vi "Get Core Group Settings.vi"(8 "error in (no error)":errorcluster, 11 "Item Ref in":T5 format="%.0x") -> (0 "error out":errorcluster, 2 "group configuration":T1={"name"="Group", "direction"=enum."Tx", "cycle timing"={"priority"=100, "decimation"=1, "offset"=0}, "timeout behavior"=enum."Increment Late Count", "enable conversion"=FALSE}, 3 "Item Ref out":T5 format="%.0x")   [LabVIEW 2017, in "DSF Shared.lvlib"]
uses:
  DSF Shared.lvlib
  <vilib>/NI Veristand/Custom Device API/Custom Device Item Ref.ctl
  DSF Core.lvlibp/Typedefs/Core Group Configuration.ctl
  DSF Core.lvlibp/Typedefs/DSF Direction.ctl
  DSF Core.lvlibp/Typedefs/DSF Timing Info.ctl
  DSF Core.lvlibp/Typedefs/DSF Timeout Behavior.ctl
  <vilib>/NI Veristand/Custom Device API/Get Item Property (Variant).vi
  <vilib>/NI Veristand/Custom Device API/Custom Device API.lvlib
  DSF Core.lvlibp
  DSF Core.lvlibp/Classes/Configuration/Core/Group/Group Configuration.lvclass
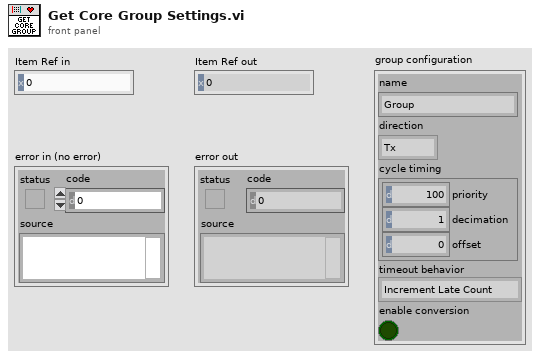
[diagram p1: front panel]
types:
  T1 = typedef "DSF Core.lvlibp/Group Configuration.lvclass/Core Group Configuration.ctl" = cluster{"name":string, "direction":T2, "cycle timing":T3, "timeout behavior":T4, "enable conversion":bool}
  T2 = typedef "DSF Core.lvlibp/DSF Direction.ctl" = enum8{"Tx", "Rx"}
  T3 = typedef "DSF Core.lvlibp/DSF Timing Info.ctl" = cluster{"priority":u64, "decimation":u64, "offset":u64}
  T4 = typedef "DSF Core.lvlibp/DSF Timeout Behavior.ctl" = enum8{"Increment Late Count", "Throw Error"}
  T5 = typedef "Custom Device API.lvlib/Custom Device Item Ref.ctl" = u64
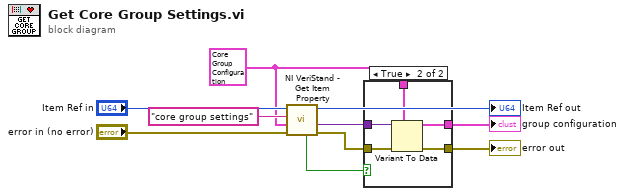
[diagram p0: block diagram]
diagram:
  w1 = T1 {"name"="Group", "direction"=enum."Tx", "cycle timing"={"priority"=100, "decimation"=1, "offset"=0}, "timeout behavior"=enum."Increment Late Count", "enable conversion"=FALSE} ("group configuration")
  n1 = call-poly <vilib>:"NI VeriStand - Get Item Property.vi"("error in (no error)"="error in (no error)", "Default Value"=w1, "Property Name"="core group settings" ("dsf options"), "Item Ref in"="Item Ref in") -> ("error out"=w9:errorcluster, "Value"=w8:variant, "Item Ref out"=→"Item Ref out":T5, "Found?"=w5:bool)  [unwired: 4 in]
  n2 = case shown="True" w5 {
    tunnel: w9 -> [w11 w17]
    tunnel: w1 -> [w12 w16]
    tunnel: w8 -> [_ w15]
    tunnel: [w11 w14] -> w7
    tunnel: [w12 w13] -> w4
    frame False {
    }
    frame True {
      n3 = Variant To Data(error in=w17, type=w16, Variant=w15) -> (data=w13:T1, error out=w14:errorcluster)
    }
  }
  "error out" <- w7
  "group configuration" <- w4
